vi "Filter Names.vi"(8 "error in (no error)":errorcluster, 9 "Name":string, 10 "Root Index":i32, 11 "Config Manager in":refnum<class "Config Manager.lvclass">) -> (0 "error out":errorcluster, 2 "Elements":refnum<class "Config Element.lvclass">[](array[class]), 3 "Config Manager out":refnum<class "Config Manager.lvclass">)   [LabVIEW 2020, in "CDM-Config.lvlib" / "Config Manager.lvclass"]
uses:
  Config Manager.lvclass
  Config Element/Config Element.lvclass
  Config Manager.lvclass/Config Manager.ctl
panel:
  out "Array":T1(array[cluster])
  out "delimited string":string
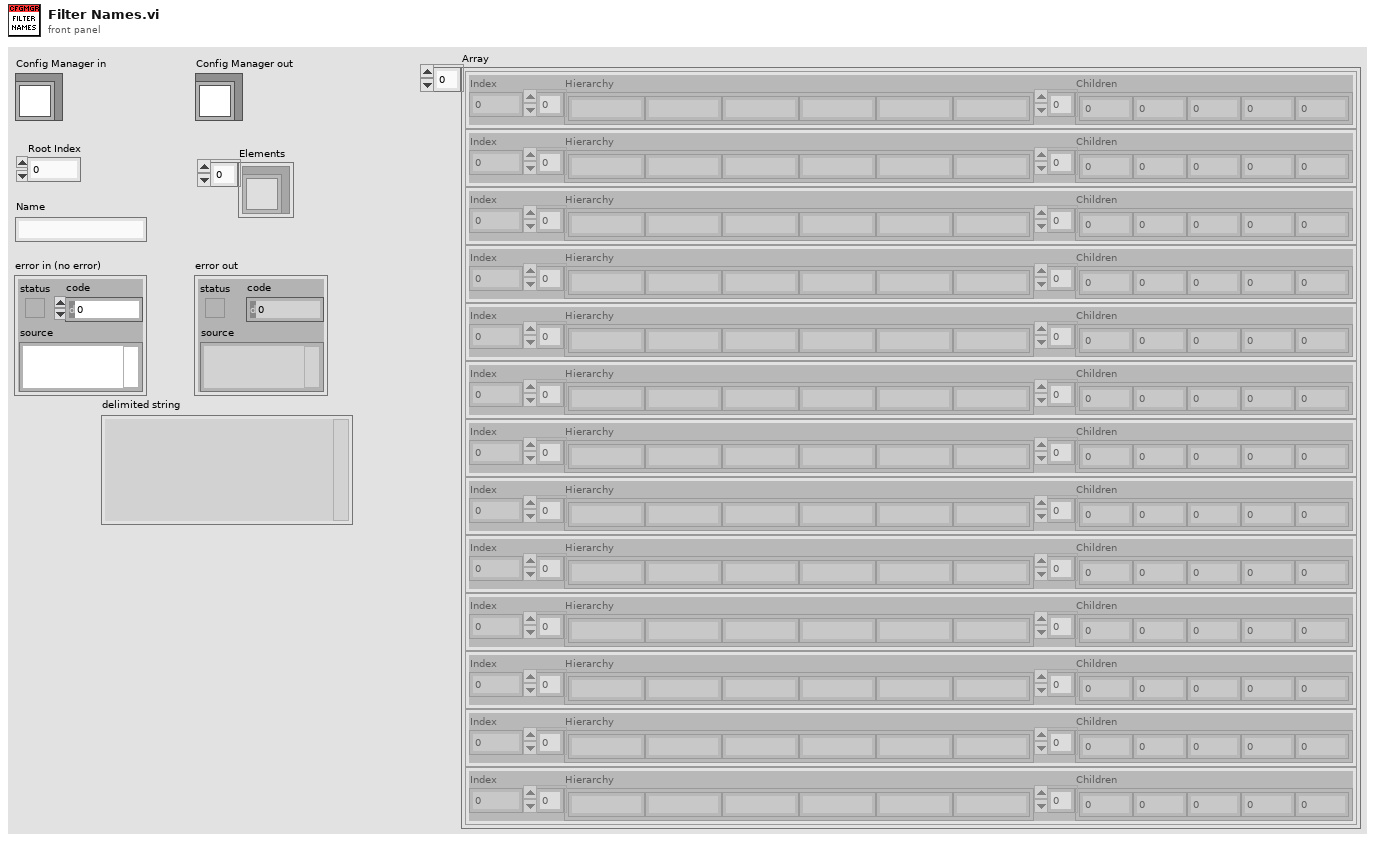
[diagram p1: front panel]
types:
  T1 = cluster{"Index":i32, "Hierarchy":string[], "Children":i32[]}[]
  T2 = typedef "CDM-Config.lvlib/Config Manager.lvclass/Ref Data.ctl" = cluster{"Elements":refnum<class "Config Element.lvclass">[], "Name Separator":string, "Hierarchy Map":map{string[], i32}, "Meta Name Map":map{string, i32[]}, "Element Map":map{refnum<class "Config Element.lvclass">, i32}, "Changed":bool[]}
  T3 = cluster{"Index":i32, "Hierarchy":string[], "Children":i32[]}
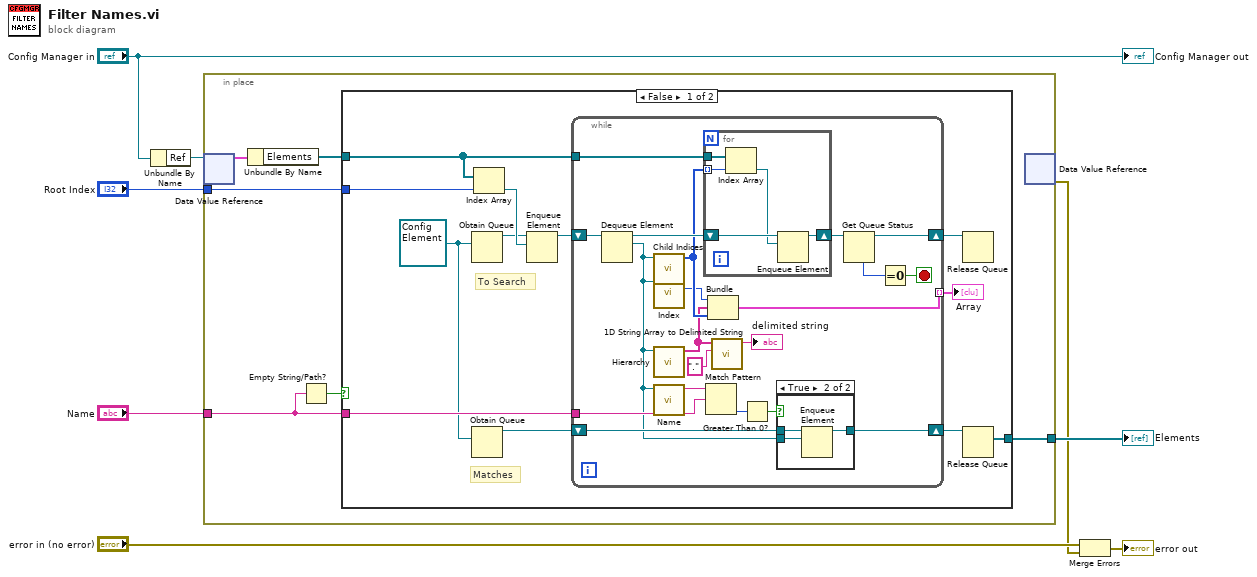
[diagram p0: block diagram]
diagram:
  n1 = Unbundle By Name("Config Manager in") -> ("Ref"=w6:refnum<data-value>)
  n2 = in-place {
    in-place-border: "Root Index" -> [w12]
    in-place-border: "Name" -> [w10]
    in-place-border: [w11] -> w2
    n3 = in-place-dvr #1(w6) -> (w14:T2)  [unwired: 1 out]
    n4 = Unbundle By Name(w14) -> ("Elements"=w13:refnum<class "Config Element.lvclass">[])
    n5 = Empty String/Path?(string/path=w10) -> (empty?=w9:bool)
    n6 = case shown="False" w9 {
      tunnel: w13 -> [w26 w56]
      tunnel: w12 -> [w25 _]
      tunnel: w10 -> [w22 _]
      tunnel: [w16 w56] -> w11
      frame False {
        w21 = refnum<class "Config Element.lvclass"> refnum ("CDM-Config.lvlib:Config Element.lvclass")
        # "Matches"
        # "To Search"
        n7 = Obtain Queue(element data type=w21) -> (queue out=w20:refnum<queue>)  [unwired: 4 in, 2 out]
        n8 = Obtain Queue(element data type=w21) -> (queue out=w19:refnum<queue>)  [unwired: 4 in, 2 out]
        n9 = Index Array(array=w26, index=w25) -> (element=w24:refnum<class "Config Element.lvclass">)
        n10 = Enqueue Element(queue=w20, element=w24) -> (queue out=w23:refnum<queue>)  [unwired: 2 in, 2 out]
        n11 = while {
          tunnel: w26 -> [w39]
          shift-right: [w36] -> w17
          shift-left: w23 -> [w46]
          shift-right: [w40] -> w18
          shift-left: w19 -> [w41]
          tunnel: w22 -> [w44]
          tunnel: [w30] -> w15 mode=indexing
          stop <- w34 stop-if-true
          n12 = Dequeue Element(queue=w46) -> (queue out=w38:refnum<queue>, element=w29:refnum<class "Config Element.lvclass">)  [unwired: 2 in, 2 out]
          n13 = call "Child Indices.vi"("Config Element in"=w29) -> ("Children"=w31:i32[])  [unwired: 9 in, 1 out]
          n14 = call "Index.vi"("Config Element in"=w29) -> ("Index"=w27:i32)  [unwired: 9 in, 1 out]
          n15 = call "Hierarchy.vi"("Config Element in"=w29) -> ("Hierarchy"=w28:string[])  [unwired: 9 in, 1 out]
          n16 = call "Name.vi"("Config Element in"=w29) -> ("Name"=w45:string)  [unwired: 9 in, 1 out]
          n17 = for {
            tunnel: w31 -> [w48] mode=indexing
            tunnel: w39 -> [w49]
            shift-right: [w50] -> w37
            shift-left: w38 -> [w51]
            n18 = Index Array(array=w49, index=w48) -> (element=w47:refnum<class "Config Element.lvclass">)
            n19 = Enqueue Element(queue=w51, element=w47) -> (queue out=w50:refnum<queue>)  [unwired: 2 in, 2 out]
          }
          n20 = Match Pattern(string=w45, regular expression=w44) -> (offset past match=w43:i32)  [unwired: 1 in, 3 out]
          n21 = Bundle("Index"=w27, "Hierarchy"=w28, "Children"=w31) -> (w30:T3)  [unwired: 1 in]
          n22 = call <vilib>:"1D String Array to Delimited String.vi"("delimiter"=".", "string array"=w28) -> ("delimited string"=→"delimited string":string)  [unwired: 9 in]
          n23 = Greater Than 0?(x=w43) -> (x > 0?=w42:bool)
          n24 = case shown="True" w42 {
            tunnel: w41 -> [w52 w55]
            tunnel: w29 -> [_ w54]
            tunnel: [w52 w53] -> w40
            frame False {
            }
            frame True {
              n25 = Enqueue Element(queue=w55, element=w54) -> (queue out=w53:refnum<queue>)  [unwired: 2 in, 2 out]
            }
          }
          n26 = Get Queue Status(queue=w37) -> (queue out=w36:refnum<queue>, # elements in queue=w35:i32)  [unwired: 2 in, 6 out]
          n27 = Equal To 0?(x=w35) -> (x = 0?=w34:bool)
        }
        "Array" <- w15
        n28 = Release Queue(queue=w17) -> ()  [unwired: 2 in, 3 out]
        n29 = Release Queue(queue=w18) -> (remaining elements=w16:refnum<class "Config Element.lvclass">[])  [unwired: 2 in, 2 out]
      }
      frame True {
      }
    }
    n30 = in-place-dvr #1() -> (w1:errorcluster)  [unwired: 1 in, 1 out]
  }
  "Elements" <- w2
  n31 = Merge Errors("error in (no error)", w1) -> (→"error out":errorcluster)
  "Config Manager out" <- "Config Manager in"
